vi "Get VIPM Dependency Map.vi"(7 "Force Reload?(F)":bool, 8 "error in":errorcluster) -> (0 "error out":errorcluster, 1 "Unmatched Packages":string[](array[string]), 2 "Internal Target Map":map{string, string}(c390), 3 "Package Array":T1[](array[typedef]))   [LabVIEW 2019]
doc: "Get paths related to all known packages and return them in a map matching them to the package name.\n\n2020-11-11: Henrik Dueholm Hansen"
uses:
  Ctl/Ctl_Package Identifier Cluster.ctl
  210f45c4-4034-4354-b09e-aea698656642.vi
  210f45c4-4034-4354-b09e-aea698656642.vi/ef9cf4bc-015b-4031-802a-4499e03f6c67.vi
  <vilib>/Utility/config.llb/NI_LVConfig.lvlib
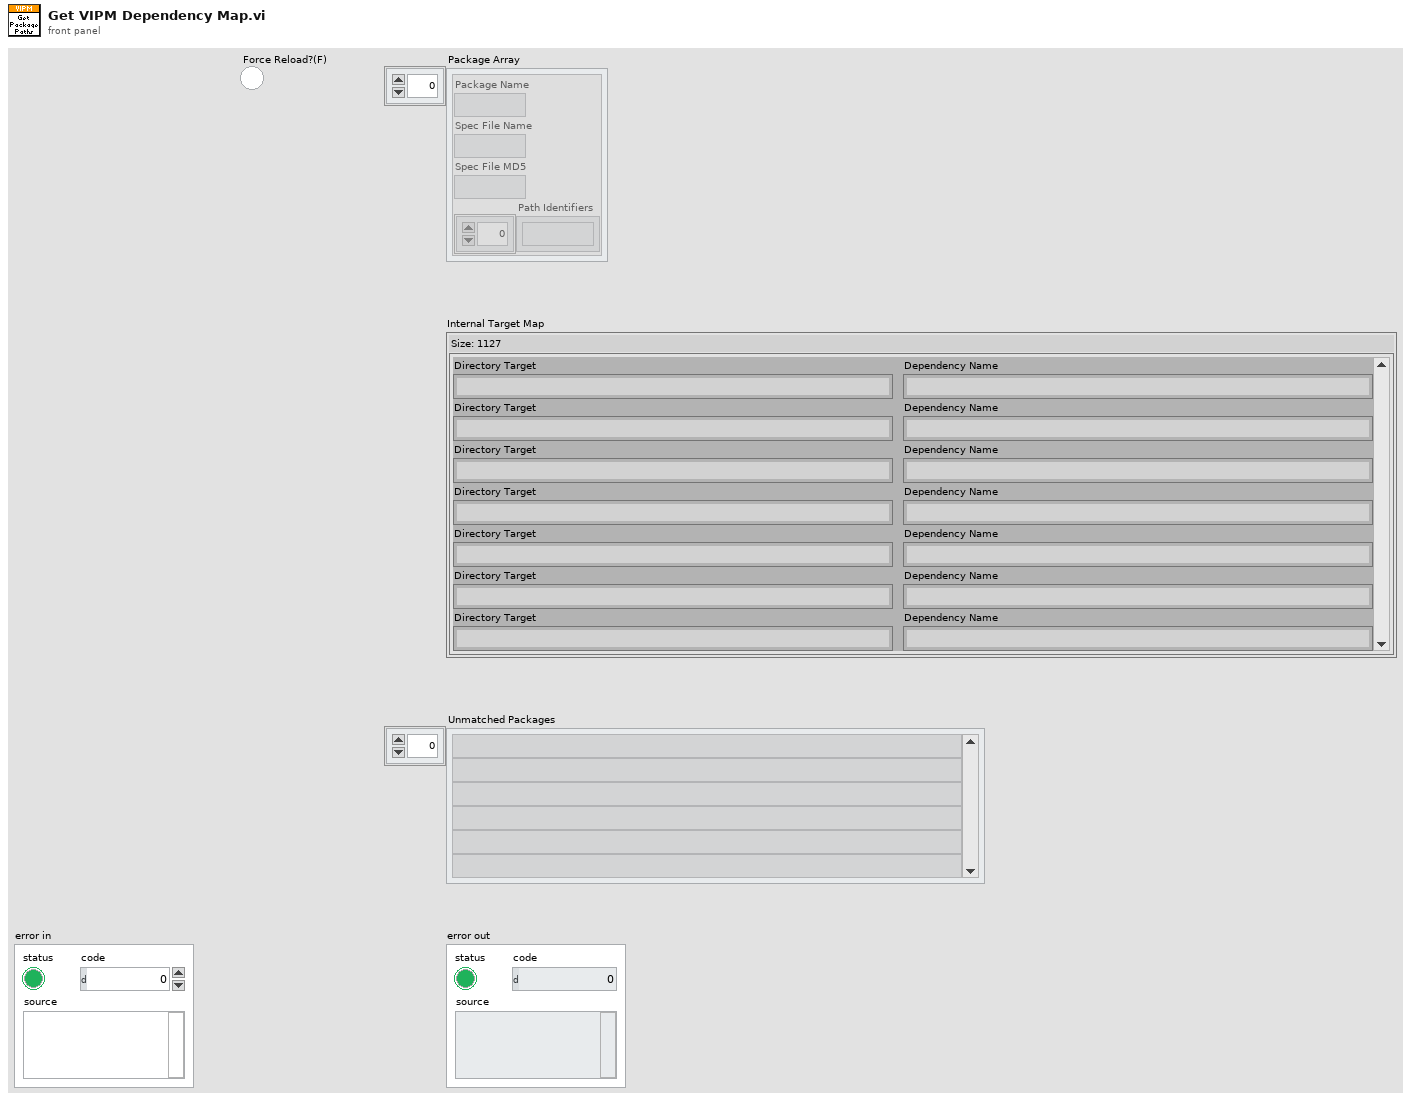
[diagram p1: front panel]
types:
  T1 = typedef "Ctl_Package Identifier Cluster.ctl" = cluster{"Package Name":string, "Spec File Name":string, "Spec File MD5":string, "Path Identifiers":string[]}
  T2 = typedef "NI_LVConfig.lvlib/Config Data RefNum.ctl" = refnum<k1>
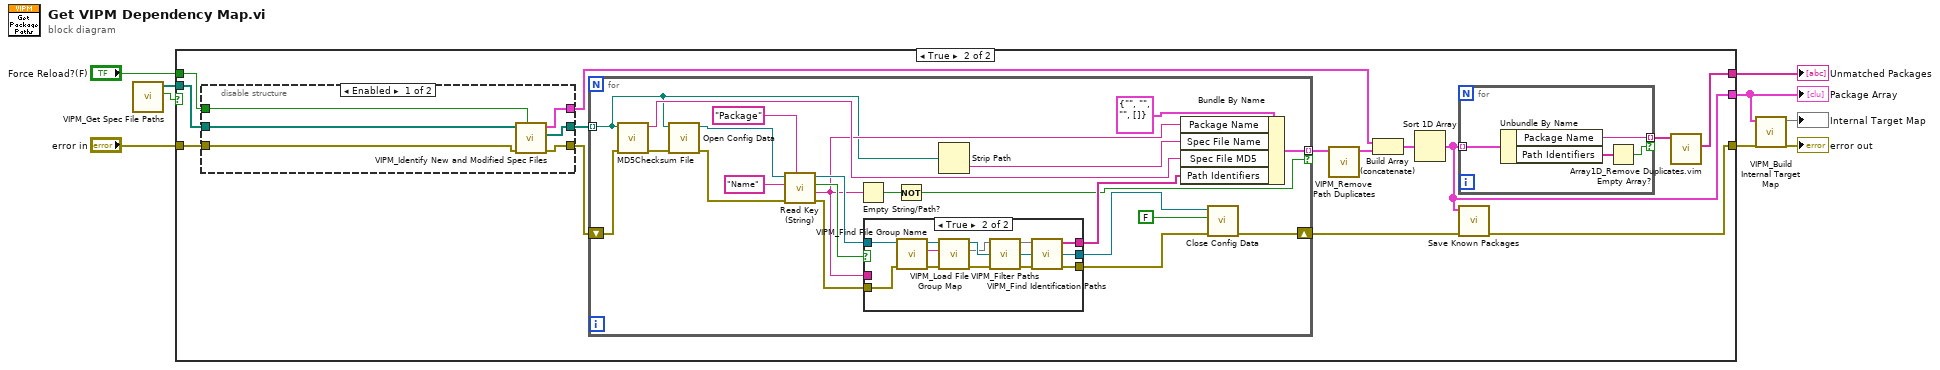
[diagram p0: block diagram]
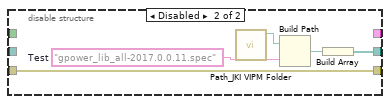
[diagram p3: hidden frame]
diagram:
  n1 = call "VIPM_Get Spec File Paths.vi"() -> ("Success?"=w3:bool, "Spec Paths"=w6:path[])  [unwired: 10 in]
  n2 = case shown="True" w3 {
    tunnel: [w9 w12] -> w7
    tunnel: "error in" -> [w9 w15]
    tunnel: w6 -> [_ w20]
    tunnel: [_ w11] -> w5
    tunnel: [_ w14] -> w4
    tunnel: "Force Reload?(F)" -> [_ w10]
    frame False {
    }
    frame True {
      n3 = disable-structure shown="Enabled" {
        disable-tunnel: w20 -> [w29 _]
        disable-tunnel: [w28 w31] -> w19
        disable-tunnel: [w27 _] -> w17
        disable-tunnel: [w26 w30] -> w16
        disable-tunnel: w15 -> [w25 w30]
        disable-tunnel: w10 -> [w24 _]
        frame Enabled {
          n4 = call "VIPM_Identify New and Modified Spec Files.vi"("Force Reload?(F)"=w24, "error in (no error)"=w25, "Spec Files"=w29) -> ("error out"=w26:errorcluster, "New or Modified Spec Files"=w28:path[], "Unchanged Package Array"=w27:T1[])  [unwired: 6 in]
        }
        frame Disabled {
          w33 = "gpower_lib_all-2017.0.0.11.spec"  # Test
          n5 = call "Path_JKI VIPM Folder.vi"() -> ("JKI\\VIPM path"=w34:path)  [unwired: 10 in, 1 out]
          n6 = Build Path(base path=w34, name or relative path=w33) -> (appended path=w32:path)
          n7 = Build Array(w32) -> (w31:path[])
        }
      }
      n8 = for {
        shift-right: [w43] -> w13
        shift-left: w16 -> [w42]
        tunnel: [w47] -> w23 mode=indexing if=w44
        tunnel: w19 -> [w40] mode=indexing
        n9 = call <vilib>:"MD5Checksum File.vi"("error in (no error)"=w42, "Path"=w40) -> ("error out"=w41:errorcluster, "MD5 message-digest"=w49:string)  [unwired: 8 in]
        n10 = call <vilib>:"Open Config Data.vi"("error in (no error)"=w41, "configuration file path"=w40) -> ("error out"=w56:errorcluster, "refnum"=w60:T2)  [unwired: 7 in, 1 out]
        n11 = call <vilib>:"Read Key (String).vi"("section"="Package", "error in (no error)"=w56, "key"="Name", "refnum"=w60) -> ("error out"=w51:errorcluster, "value"=w46:string, "found?"=w57:bool, "refnum out"=w55:T2)  [unwired: 4 in]
        n12 = Empty String/Path?(string/path=w46) -> (empty?=w45:bool)
        n13 = case shown="True" w57 {
          tunnel: w55 -> [w62 w72]
          tunnel: [w62 w68] -> w54
          tunnel: [w61 w67] -> w52
          tunnel: w51 -> [w61 w71]
          tunnel: w46 -> [_ _]
          tunnel: [_ w63] -> w48
          frame False {
          }
          frame True {
            n14 = call "VIPM_Find File Group Name.vi"("error in (no error)"=w71, "Refnum in"=w72) -> ("error out"=w69:errorcluster, "File Group Name"=w66:string, "Refnum out"=w70:T2)  [unwired: 7 in]
            n15 = call "VIPM_Load File Group Map.vi"("error in (no error)"=w69, "File Group Name"=w66, "Refnum in"=w70) -> ("error out"=w67:errorcluster, "Ordered File Group map"=w64:map{string, string[]}, "Refnum out"=w68:T2)  [unwired: 6 in]
            n16 = call "VIPM_Filter Paths.vi"("Unfiltered map in"=w64) -> ("Filtered map out"=w65:map{string, string[]})  [unwired: 10 in]
            n17 = call "VIPM_Find Identification Paths.vi"("Filtered map in"=w65) -> ("Found Identification Paths"=w63:string[])  [unwired: 10 in]
          }
        }
        n18 = Not(x=w45) -> (.not. x?=w44:bool)
        n19 = Strip Path(path=w40) -> (name=w39:string)  [unwired: 1 out]
        n20 = Bundle By Name(cluster=T1 {"Package Name"="", "Spec File Name"="", "Spec File MD5"="", "Path Identifiers"=[]}, "Package Name"=w46, "Spec File Name"=w39, "Spec File MD5"=w49, "Path Identifiers"=w48) -> (w47:T1)
        n21 = call <vilib>:"Close Config Data.vi"("error in (no error)"=w52, "write file if changed (T)"=FALSE, "refnum"=w54) -> ("error out"=w43:errorcluster)  [unwired: 7 in, 1 out]
      }
      n22 = call "VIPM_Remove Path Duplicates.vi"("Package Array in"=w23) -> ("Package Array out"=w22:T1[])  [unwired: 10 in]
      n23 = Build Array (concatenate)(w17, w22) -> (w18:T1[])
      n24 = Sort 1D Array(array=w18) -> (sorted array=w14:T1[])
      n25 = for {
        tunnel: w14 -> [w38] mode=indexing
        tunnel: [w36] -> w21 mode=indexing if=w35
        n26 = Unbundle By Name(w38) -> ("Package Name"=w36:string, "Path Identifiers"=w37:string[])
        n27 = Empty Array?(array=w37) -> (empty?=w35:bool)
      }
      n28 = call "Save Known Packages.vi"("error in (no error)"=w13, "Package Array from File"=w14) -> ("error out"=w12:errorcluster)  [unwired: 8 in, 1 out]
      n29 = call "Array1D_Remove Duplicates.vim"("Array"=w21) -> ("Sorted Removed duplicates"=w11:string[])  [unwired: 8 in, 2 out]
    }
  }
  "error out" <- w7
  "Unmatched Packages" <- w5
  "Package Array" <- w4
  n30 = call "VIPM_Build Internal Target Map.vi"("Package Array"=w4) -> ("Internal Target Map"=→"Internal Target Map":map{string, string})  [unwired: 10 in]
